vi "Line Minimum Fletcher.vi"(6 "Parsed Formula":cluster{"table":i32[][], "result":dbl[]}, 7 "Variables":i32[](array[numeric])=[0, 0], 8 "zeps":dbl=1e-12 format="%.2e", 9 "tol":dbl=1e-06 format="%.2e", 10 "p":dbl[](array[numeric]) format="%.2f", 11 "xit":dbl[](array[numeric]) format="%.2f") -> (0 "error":i32, 1 "f(p)":dbl format="%.2f", 2 "pnew":dbl[](array[numeric]) format="%.2f", 3 "xitnew":dbl[](array[numeric]) format="%.2f")   [LabVIEW 2014, in "NI_Gmath.lvlib"]
uses:
  NI_Gmath.lvlib
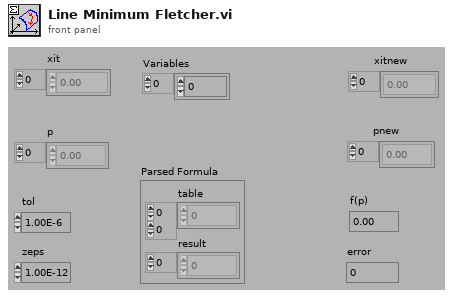
[diagram p1: front panel]
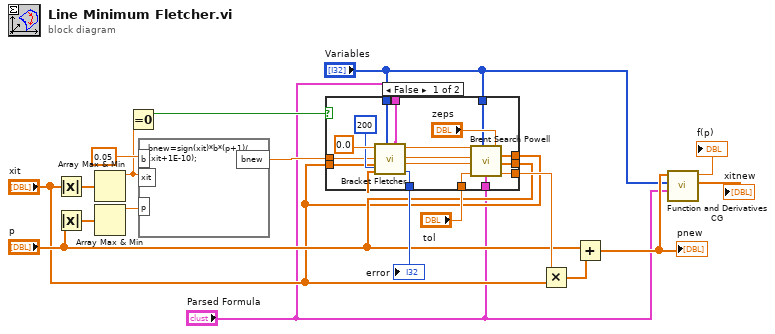
[diagram p0: block diagram]
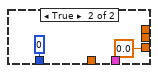
[diagram p2: hidden frame]
diagram:
  n1 = Absolute Value(x="xit") -> (abs(x)=w10:dbl[])
  n2 = Absolute Value(x="p") -> (abs(x)=w9:dbl[])
  n3 = Array Max & Min(array=w10) -> (max value=w5:dbl)  [unwired: 3 out]
  n4 = Array Max & Min(array=w9) -> (max value=w8:dbl)  [unwired: 3 out]
  n5 = Equal To 0?(x=w5) -> (x = 0?=w3:bool)
  n6 = formula code="bnew=sign(xit)*b*(p+1)/(xit+1E-10);"("b"=0.05, "xit"=w5, "p"=w8) -> ("bnew"=w6:dbl)
  n7 = case shown="False" w3 {
    tunnel: w6 -> [w33 _]
    tunnel: "xit" -> [w24 _]
    tunnel: "p" -> [w32 _]
    tunnel: [w31 0.0] -> w16
    tunnel: "tol" -> [w29 _]
    tunnel: [w25 0] -> w18
    tunnel: "xit" -> [w23 _]
    tunnel: "Parsed Formula" -> [w22 _]
    tunnel: "Variables" -> [w21 _]
    tunnel: "Variables" -> [w20 _]
    tunnel: "Parsed Formula" -> [w19 _]
    frame False {
      n8 = call "Bracket Fletcher.vi"("Parsed Formula"=w19, "loops"=u32 200, "Variables"=w20, "p"=w32, "xit"=w23, "b (start)"=w33, "a (start)"=0.0) -> ("error"=w25:i32, "c (bracket)"=w28:dbl, "b (bracket)"=w27:dbl, "a (bracket)"=w26:dbl)  [unwired: 1 in]
      n9 = call "Brent Search Powell.vi"("p"=w32, "xit"=w24, "ZEPS"="zeps", "Parsed Formula"=w22, "Variables"=w21, "tol"=w29, "c (start)"=w28, "b (start)"=w27, "a (start)"=w26) -> ("u"=w31:dbl)  [unwired: 2 in]
    }
    frame True {
    }
  }
  "error" <- w18
  n10 = Multiply(x=w16, y="xit") -> (x*y=w13:dbl[])
  n11 = Add(x="p", y=w13) -> (x+y=w15:dbl[])
  "pnew" <- w15
  n12 = call "Function and Derivatives CG.vi"("Parsed Formula"="Parsed Formula", "Variables"="Variables", "X"=w15) -> ("df/dX"=→"xitnew":dbl[], "f(X)"=→"f(p)":dbl)  [unwired: 7 in]
